vi "ViperHawk Plot Setup.vi"(7 "Plot File":T1, 8 "error in (no error)":errorcluster, 11 "Log Inverter File":path) -> (0 "error out":errorcluster, 2 "Data with 0's and 1's":dbl[][](array[numeric]), 3 "Time Stamp":timestamp[](array[timestamp]), 4 "Y-Axis Search":string[](array[string]), 6 "Y-Axis Drop Down Data":string[](array[string]))   [LabVIEW 2016]
uses:
  Type Definitions/ViperHawk/ViperHawk Plot File.ctl
  <vilib>/Utility/file.llb/Read From Spreadsheet File (string).vi
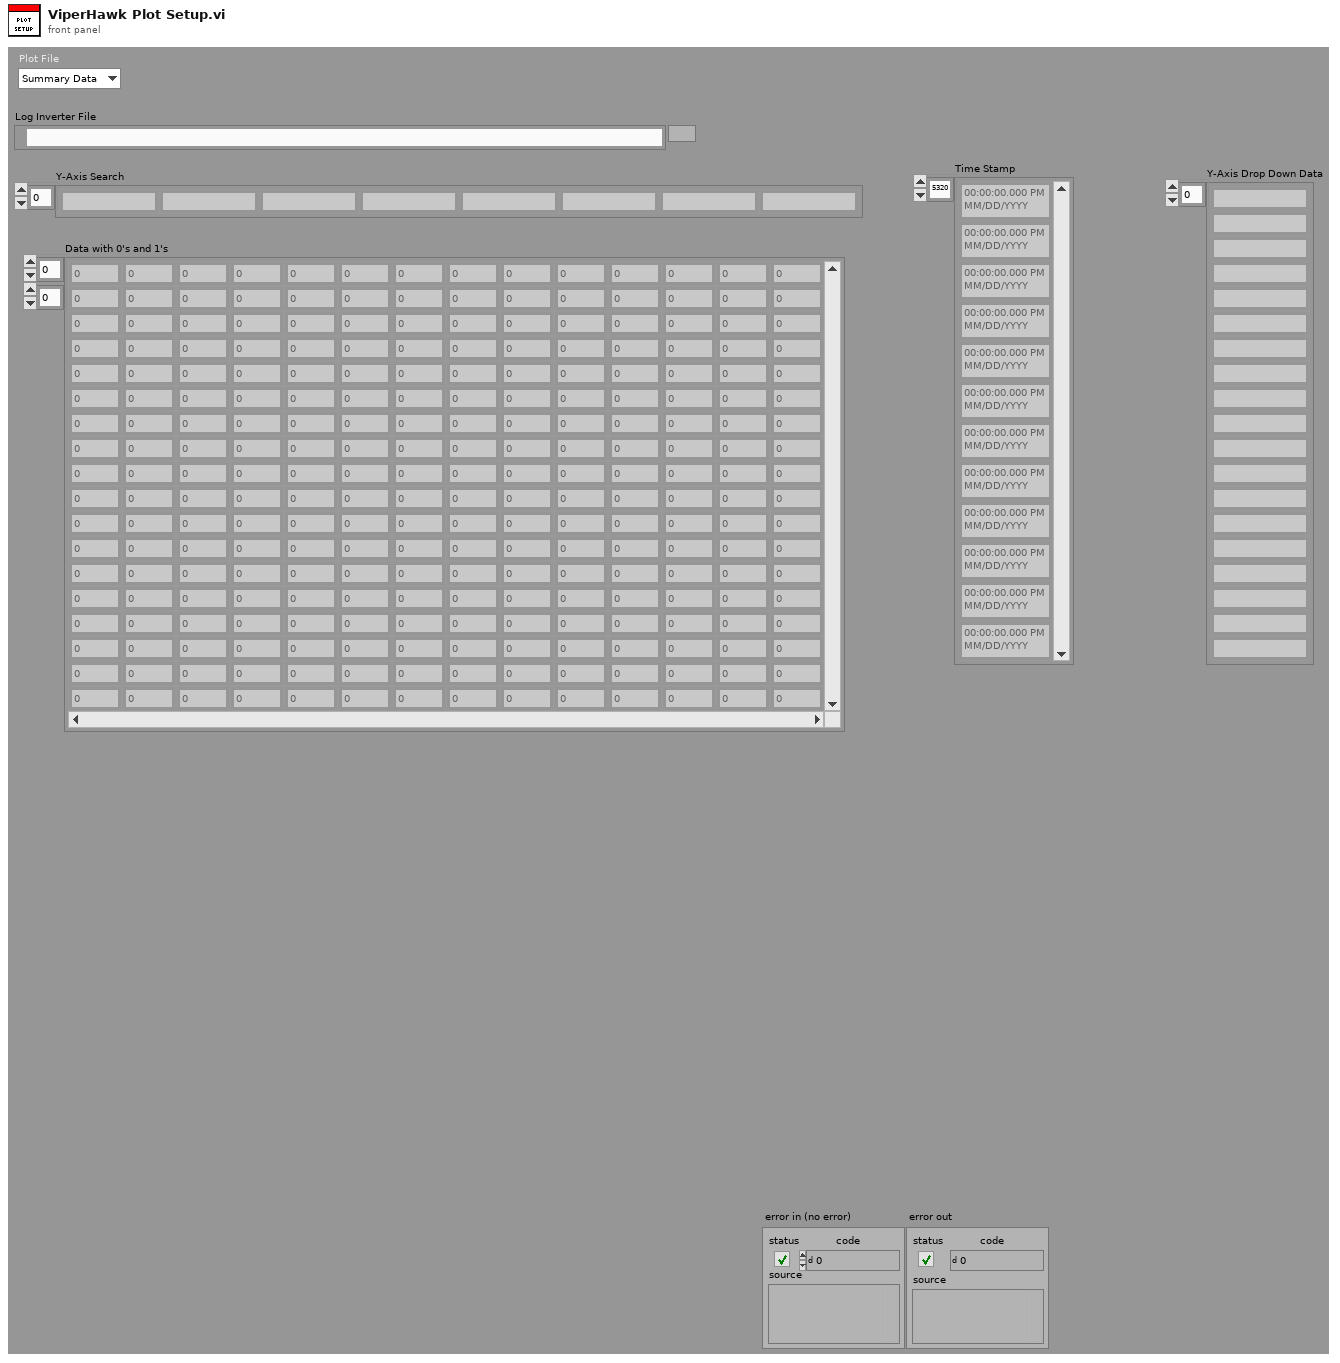
[diagram p1: front panel]
types:
  T1 = typedef "ViperHawk Plot File.ctl" = enum16{"Summary Data"}
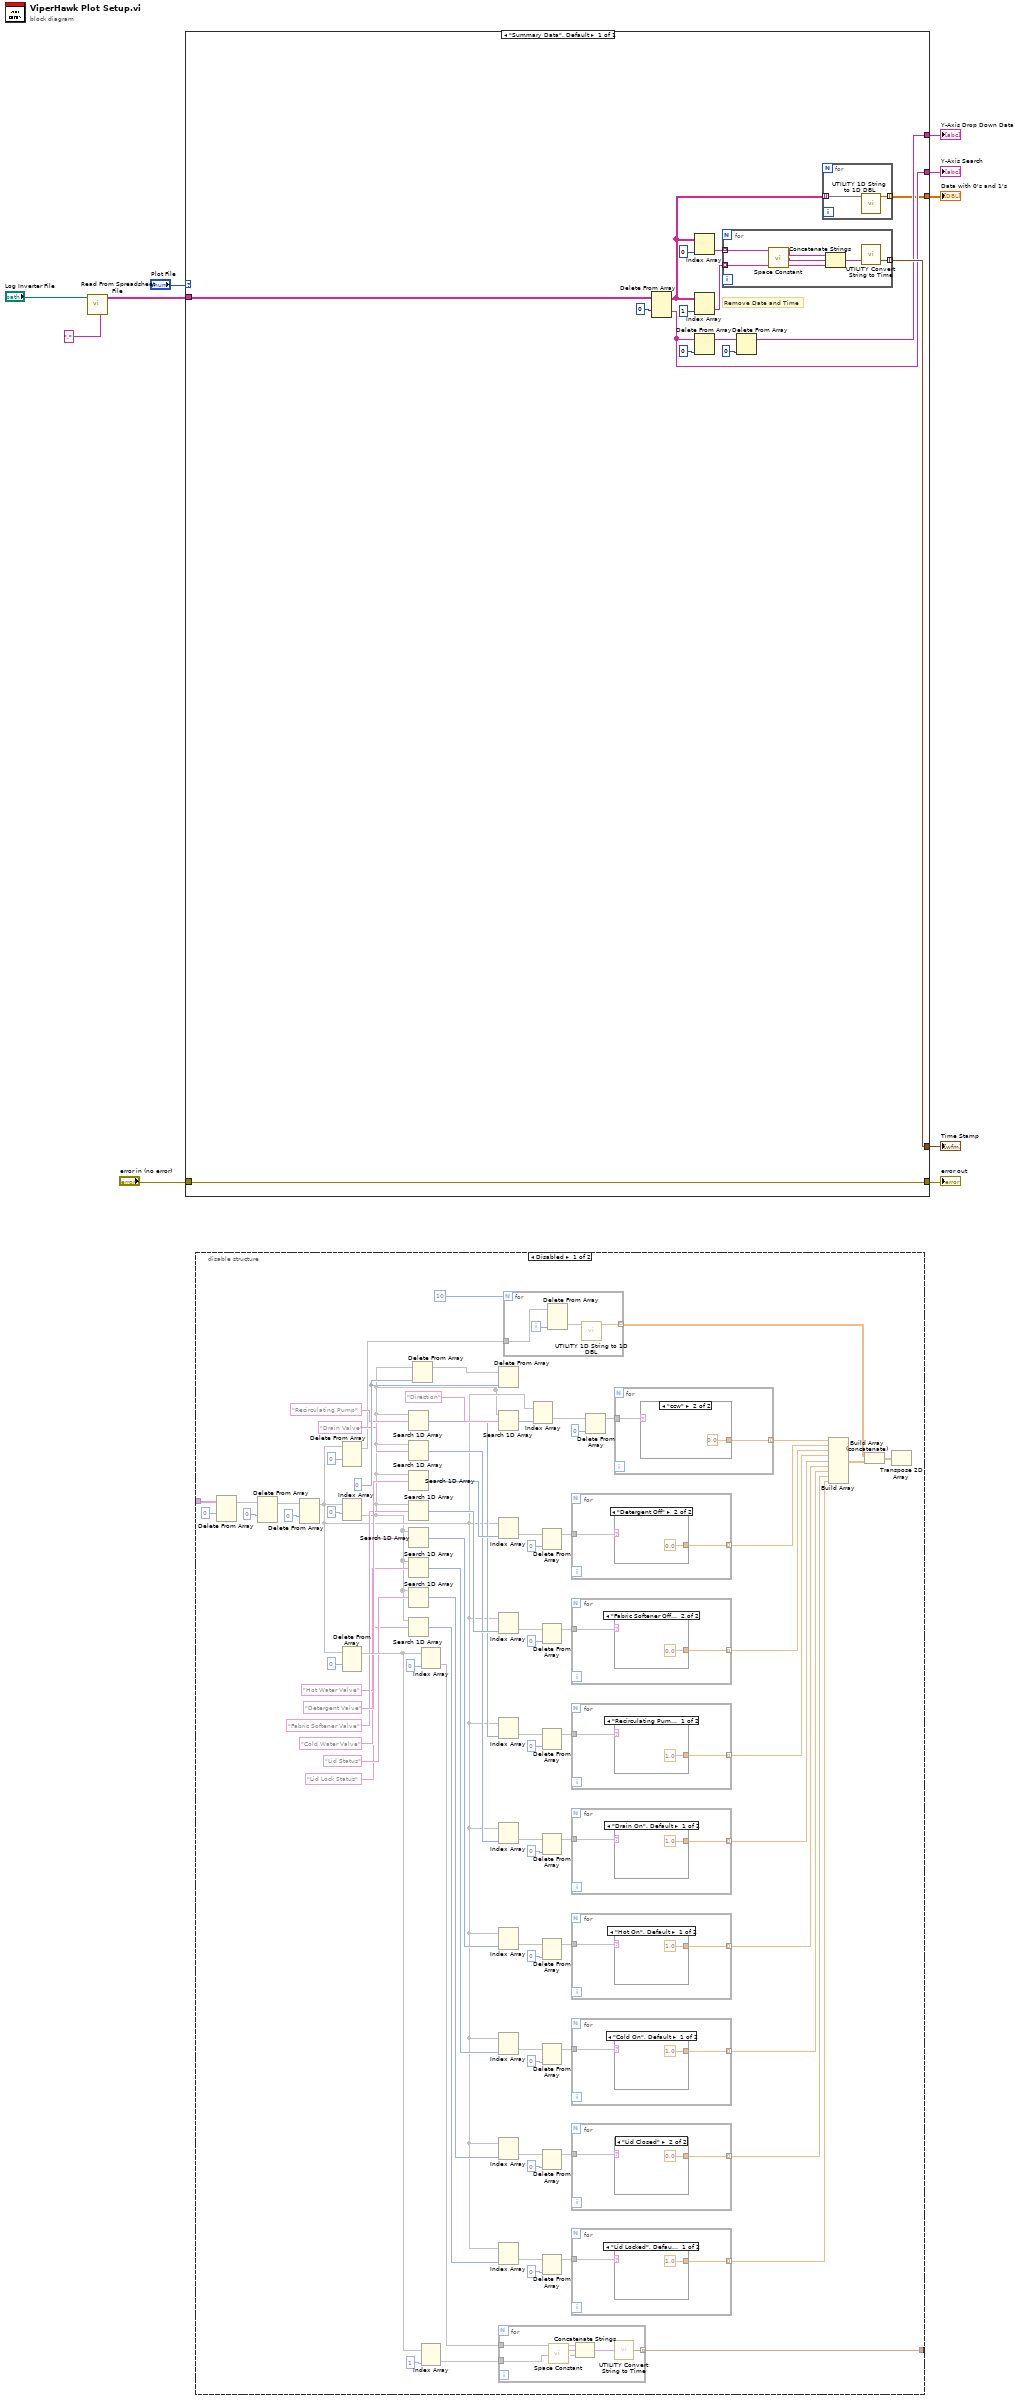
[diagram p0: block diagram]
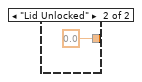
[diagram p2: hidden frame]
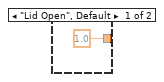
[diagram p3: hidden frame]
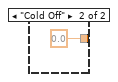
[diagram p4: hidden frame]
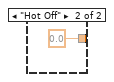
[diagram p5: hidden frame]
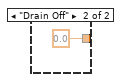
[diagram p6: hidden frame]
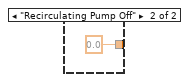
[diagram p7: hidden frame]
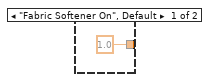
[diagram p8: hidden frame]
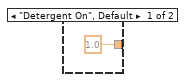
[diagram p9: hidden frame]
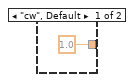
[diagram p10: hidden frame]
diagram:
  n1 = call-poly <vilib>:"Read From Spreadsheet File.vi"("delimiter (\\t)"="," ("delimiter (\\t)"), "file path (dialog if empty)"="Log Inverter File") -> ("all rows"=w8:string[][])  [unwired: 5 in, 4 out]
  n2 = case shown="\"Summary Data\", Default" "Plot File" {
    tunnel: w8 -> [w19]
    tunnel: [w11] -> w1
    tunnel: "error in (no error)" -> [w25]
    tunnel: [w25] -> w5
    tunnel: [w20] -> w4
    tunnel: [w13] -> w3
    tunnel: [w17] -> w2
    frame "Summary Data", Default {
      # "Remove Date and Time"
      n3 = Delete From Array(array=w19, index (row)=0) -> (deleted portion=w17:string[], array with subset deleted=w12:string[][])  [unwired: 2 in]
      n4 = Index Array(array=w12, index (col)=0 ("disabled index (col)")) -> (element=w22:string[])  [unwired: 1 in]
      n5 = Index Array(array=w12, index (col)=1 ("disabled index (col)")) -> (element=w21:string[])  [unwired: 1 in]
      n6 = Delete From Array(array=w17, index=0) -> (array with subset deleted=w16:string[])  [unwired: 1 in, 1 out]
      n7 = for {
        tunnel: w21 -> [w31] mode=indexing
        tunnel: w22 -> [w30] mode=indexing
        tunnel: [w29] -> w20 mode=indexing
        n8 = call <vilib>:"Space Constant.vi"() -> ("String"=w32:string)
        n9 = Concatenate Strings(w30, w32, w31) -> (w28:string)
        n10 = call "UTILITY Convert String to Time.vi"("date/time string"=w28) -> ("Resulting Time Stamp"=w29:timestamp)  [unwired: 8 in, 2 out]
      }
      n11 = Delete From Array(array=w16, index=0) -> (array with subset deleted=w13:string[])  [unwired: 1 in, 1 out]
      n12 = for {
        tunnel: w12 -> [w26] mode=indexing
        tunnel: [w27] -> w11 mode=indexing
        n13 = call "UTILITY 1D String to 1D DBL.vi"("Save Data"=w26) -> ("DBL"=w27:dbl[])  [unwired: 10 in]
      }
    }
  }
  "error out" <- w5
  "Time Stamp" <- w4
  "Y-Axis Drop Down Data" <- w3
  "Y-Axis Search" <- w2
  "Data with 0's and 1's" <- w1
  n14 = disable-structure shown="Disabled" {
    disable-tunnel: _ -> [w112 _]
    disable-tunnel: [w36 _] -> _
    frame Disabled {
      w109 = 0 ("index")
      n15 = Delete From Array(array=w112, index (row)=0) -> (array with subset deleted=w42)  [unwired: 2 in, 1 out]
      n16 = Delete From Array(array=w42, index (row)=0) -> (array with subset deleted=w41)  [unwired: 2 in, 1 out]
      n17 = Delete From Array(array=w41, index (row)=0) -> (array with subset deleted=w37)  [unwired: 2 in, 1 out]
      n18 = Delete From Array(array=w37, index (row)=0) -> (array with subset deleted=w43)  [unwired: 2 in, 1 out]
      n19 = Index Array(array=w37, index (row)=0 ("disabled index (col)")) -> (element=w34)  [unwired: 1 in]
      n20 = Delete From Array(array=w37, index (row)=0) -> (array with subset deleted=w111)  [unwired: 2 in, 1 out]
      n21 = Search 1D Array(1D array=w34, element="Recirculating Pump") -> (index of element=w84:i32)  [unwired: 1 in]
      n22 = Search 1D Array(1D array=w34, element="Drain Valve") -> (index of element=w82:i32)  [unwired: 1 in]
      n23 = Search 1D Array(1D array=w34, element="Detergent Valve") -> (index of element=w94:i32)  [unwired: 1 in]
      n24 = Search 1D Array(1D array=w34, element="Fabric Softener Valve") -> (index of element=w92:i32)  [unwired: 1 in]
      n25 = Search 1D Array(1D array=w34, element="Hot Water Valve") -> (index of element=w73:i32)  [unwired: 1 in]
      n26 = Search 1D Array(1D array=w34, element="Cold Water Valve") -> (index of element=w72:i32)  [unwired: 1 in]
      n27 = Search 1D Array(1D array=w34, element="Lid Status") -> (index of element=w63:i32)  [unwired: 1 in]
      n28 = Search 1D Array(1D array=w34, element="Lid Lock Status") -> (index of element=w62:i32)  [unwired: 1 in]
      n29 = Delete From Array(array=w34, index=w109) -> (array with subset deleted=w108)  [unwired: 1 in, 1 out]
      n30 = Index Array(array=w111, index (col)=0 ("disabled index (col)")) -> (element=w107)  [unwired: 1 in]
      n31 = Index Array(array=w111, index (col)=1 ("disabled index (col)")) -> (element=w106)  [unwired: 1 in]
      n32 = Delete From Array(array=w108, index=w109) -> (array with subset deleted=w35)  [unwired: 1 in, 1 out]
      n33 = Search 1D Array(1D array=w34, element="Direction") -> (index of element=w101:i32)  [unwired: 1 in]
      n34 = Index Array(array=w37, index (col)=w94) -> (element=w95)  [unwired: 1 in]
      n35 = Index Array(array=w37, index (col)=w92) -> (element=w91)  [unwired: 1 in]
      n36 = Index Array(array=w37, index (col)=w84) -> (element=w85)  [unwired: 1 in]
      n37 = Index Array(array=w37, index (col)=w82) -> (element=w81)  [unwired: 1 in]
      n38 = Index Array(array=w37, index (col)=w73) -> (element=w74)  [unwired: 1 in]
      n39 = Index Array(array=w37, index (col)=w72) -> (element=w71)  [unwired: 1 in]
      n40 = Index Array(array=w37, index (col)=w63) -> (element=w64)  [unwired: 1 in]
      n41 = Index Array(array=w37, index (col)=w62) -> (element=w61)  [unwired: 1 in]
      n42 = for {
        tunnel: w106 -> [w116]
        tunnel: w107 -> [w115]
        tunnel: [w114] -> w36 mode=indexing
        n43 = call <vilib>:"Space Constant.vi"() -> ("String"=w117:string)
        n44 = Concatenate Strings(w115, w117, w116) -> (w113:string)
        n45 = call "UTILITY Convert String to Time.vi"("date/time string"=w113) -> ("Resulting Time Stamp"=w114:timestamp)
      }
      n46 = for {
        N: 10 -> [_]
        tunnel: w43 -> [w121]
        tunnel: [w118] -> w46 mode=indexing
        i -> [w120]
        n47 = Delete From Array(array=w121, index (col)=w120) -> (deleted portion=w119)  [unwired: 2 in, 1 out]
        n48 = call "UTILITY 1D String to 1D DBL.vi"("Save Data"=w119) -> ("DBL"=w118:dbl[])  [unwired: 10 in]
      }
      n49 = Index Array(array=w37, index (col)=w101) -> (element=w100)  [unwired: 1 in]
      n50 = Delete From Array(array=w95, index=0) -> (array with subset deleted=w93)  [unwired: 1 in, 1 out]
      n51 = Delete From Array(array=w91, index=0) -> (array with subset deleted=w88)  [unwired: 1 in, 1 out]
      n52 = Delete From Array(array=w85, index=0) -> (array with subset deleted=w83)  [unwired: 1 in, 1 out]
      n53 = Delete From Array(array=w81, index=0) -> (array with subset deleted=w78)  [unwired: 1 in, 1 out]
      n54 = Delete From Array(array=w74, index=0) -> (array with subset deleted=w77)  [unwired: 1 in, 1 out]
      n55 = Delete From Array(array=w71, index=0) -> (array with subset deleted=w68)  [unwired: 1 in, 1 out]
      n56 = Delete From Array(array=w64, index=0) -> (array with subset deleted=w67)  [unwired: 1 in, 1 out]
      n57 = Delete From Array(array=w61, index=0) -> (array with subset deleted=w58)  [unwired: 1 in, 1 out]
      n58 = for {
        tunnel: w93 -> [w151]
        tunnel: [w150] -> w56 mode=indexing
        n59 = case shown="\"Detergent Off\"" w151 {
          tunnel: [1.0 0.0] -> w150
          frame "Detergent On", Default {
          }
          frame "Detergent Off" {
          }
        }
      }
      n60 = for {
        tunnel: w88 -> [w147]
        tunnel: [w146] -> w55 mode=indexing
        n61 = case shown="\"Fabric Softener Off\"" w147 {
          tunnel: [1.0 0.0] -> w146
          frame "Fabric Softener On", Default {
          }
          frame "Fabric Softener Off" {
          }
        }
      }
      n62 = for {
        tunnel: w83 -> [w143]
        tunnel: [w142] -> w54 mode=indexing
        n63 = case shown="\"Recirculating Pump On\", Default" w143 {
          tunnel: [1.0 0.0] -> w142
          frame "Recirculating Pump On", Default {
          }
          frame "Recirculating Pump Off" {
          }
        }
      }
      n64 = for {
        tunnel: w78 -> [w139]
        tunnel: [w138] -> w53 mode=indexing
        n65 = case shown="\"Drain On\", Default" w139 {
          tunnel: [1.0 0.0] -> w138
          frame "Drain On", Default {
          }
          frame "Drain Off" {
          }
        }
      }
      n66 = for {
        tunnel: w77 -> [w135]
        tunnel: [w134] -> w52 mode=indexing
        n67 = case shown="\"Hot On\", Default" w135 {
          tunnel: [1.0 0.0] -> w134
          frame "Hot On", Default {
          }
          frame "Hot Off" {
          }
        }
      }
      n68 = for {
        tunnel: w68 -> [w131]
        tunnel: [w130] -> w51 mode=indexing
        n69 = case shown="\"Cold On\", Default" w131 {
          tunnel: [1.0 0.0] -> w130
          frame "Cold On", Default {
          }
          frame "Cold Off" {
          }
        }
      }
      n70 = for {
        tunnel: w67 -> [w127]
        tunnel: [w126] -> w50 mode=indexing
        n71 = case shown="\"Lid Closed\"" w127 {
          tunnel: [1.0 0.0] -> w126
          frame "Lid Open", Default {
          }
          frame "Lid Closed" {
          }
        }
      }
      n72 = for {
        tunnel: w58 -> [w123]
        tunnel: [w122] -> w49 mode=indexing
        n73 = case shown="\"Lid Locked\", Default" w123 {
          tunnel: [1.0 0.0] -> w122
          frame "Lid Locked", Default {
          }
          frame "Lid Unlocked" {
          }
        }
      }
      n74 = Delete From Array(array=w100, index=0) -> (array with subset deleted=w98)  [unwired: 1 in, 1 out]
      n75 = for {
        tunnel: w98 -> [w155]
        tunnel: [w154] -> w57 mode=indexing
        n76 = case shown="\"ccw\"" w155 {
          tunnel: [1.0 0.0] -> w154
          frame "cw", Default {
          }
          frame "ccw" {
          }
        }
      }
      n77 = Build Array(w57, w56, w55, w54, w53, w52, w51, w50, w49) -> (w47:dbl[][])
      n78 = Build Array (concatenate)(w46, w47) -> (w45:dbl[][])
      n79 = Transpose 2D Array(2D array=w45) -> (transposed array=w33:dbl[][])
    }
    frame Enabled {
    }
  }
